vi "StandAlone_CloseSessions.vi"() -> ()   [LabVIEW 2019]
panel:
  in  "instrument handle 3":refnum<k15>
  in  "instrument handle 2":refnum<k15> caption="instrument handle"
  in  "instrument handle":refnum<k15>
  in  "VISA resource name":refnum<visa-resource-name>
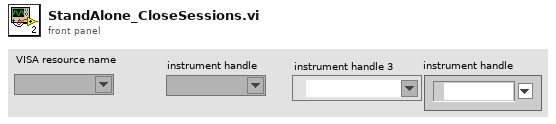
[diagram p1: front panel]
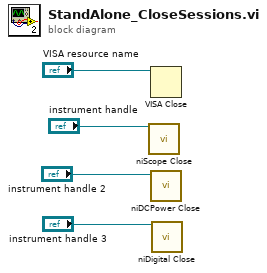
[diagram p0: block diagram]
diagram:
  n1 = call <instrlib>:"niScope Close.vi"("instrument handle"="instrument handle") -> ()  [unwired: 14 in, 1 out]
  n2 = VISA Close(VISA resource name="VISA resource name") -> ()  [unwired: 1 in, 1 out]
  n3 = call <instrlib>:"niDCPower Close.vi"("instrument handle"="instrument handle 2") -> ()  [unwired: 10 in, 1 out]
  n4 = call <instrlib>:"niDigital Close.vi"("instrument handle"="instrument handle 3") -> ()  [unwired: 14 in, 1 out]
